vi "Acquisition Message Loop.vi"(6 "Data-Chart-Reference":refnum<vi>, 8 "error in (no error)":errorcluster, 9 "Data Queue":refnum<queue>, 10 "Data Notifier":refnum<notifier>, 11 "Message Queues":T1) -> (0 "error out":errorcluster)   [LabVIEW 2018, in "Acquisition.lvlib"]
doc: "Message loop for handling messages pertaining to the acquisition of data from the hardware."
uses:
  Acquisition.lvlib
  support/Message Queue/All Message Queues.ctl
  support/Message Queue/Message Cluster.ctl
  Hardware Configuration.ctl
  Acquisition State.ctl
  <vilib>/Platform/TimedLoop/XDataNode/timing_clust.ctl
  <vilib>/Platform/TimedLoop/XDataNode/nitl_modes.ctl
  <vilib>/Platform/TimedLoop/XDataNode/wakeup.ctl
  support/Message Queue/Enqueue Message (Single).vi
  <vilib>/Utility/error.llb/Error Cluster From Error Code.vi
  <vilib>/platform/TimedLoop/XDataNode/XDataNode.xnode
  <vilib>/ErrorRing/Error Ring.xnode
  support/Message Queue/Message Queue.lvlib
  <vilib>/Platform/TimedLoop/XDataNode/XDNodeRunTimeDep.lvlib
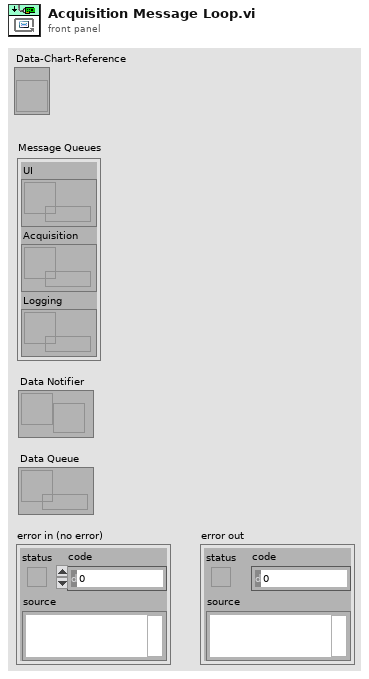
[diagram p1: front panel]
types:
  T1 = typedef "Message Queue.lvlib/All Message Queues.ctl" = cluster{"UI":refnum<queue>, "Acquisition":refnum<queue>, "Logging":refnum<queue>}
  T2 = typedef "Acquisition.lvlib/Hardware Configuration.ctl" = cluster{"DAQmx Channel 1":tag, "DAQmx Channel 2":tag, "DAQmx Channel 3":tag, "Channel 1 Name":string, "Channel 2 Name":string, "Channel 3 Name":string, "Input Config Channel 1":i32, "Input Config Channel 2":i32, "Input Config Channel 3":i32, "Offset Channel 1":dbl, "Offset Channel 2":dbl, "Offset Channel 3":dbl, "Scale Channel 1":dbl, "Scale Channel 2":dbl, "Scale Channel 3":dbl, "DAQmx Counter Channel":tag, "Counter Name":string, "Sample time":u32, "Samples per second":dbl, "Sample mode":u16, "Samples per channel":i32, "DAQmx AI Task":refnum<k21>, "DAQmx Counter Task":refnum<k21>}
  T3 = typedef "XDNodeRunTimeDep.lvlib/timing_clust.ctl" = cluster{"Expected End [f-1]":u64, "Actual End [f-1]":u64, "Finished Late? [f-1]":bool, "Expected End [i-1]":u64, "Actual End [i-1]":u64, "Finished Late? [i-1]":bool, "Expected Start [i]":u64, "Actual Start [i]":u64, "Expected Start [f]":u64, "Actual Start [f]":u64, "Source Name":string, "Structure Name":string, "Period":i64, "Deadline":i64, "Offset":i64, "Start":i64, "Priority":i32, "Timeout":i32, "Mode":T4, "Wakeup Reason":T5, "Error":errorcluster, "Source Type":string, "Secondary Source Type":string, "Global End Time":u64, "Global Start Time":u64, "Frame Duration":u64, "Iteration Duration":u64, "Assigned CPU":i32, "I/O Scan Engine Mode":u32}
  T4 = typedef "XDNodeRunTimeDep.lvlib/nitl_modes.ctl" = enum32{"No Change", "Process missed periods, maintain original phase", "Discard missed periods, maintain original phase", "Process missed periods, ignore original phase", "Discard missed periods, ignore original phase"}
  T5 = typedef "XDNodeRunTimeDep.lvlib/wakeup.ctl" = enum32{"Normal", "Aborted", "Asynchronous wakeup", "Timing source error", "Timed loop error", "Timeout"}
  T6 = typedef "Acquisition.lvlib/Acquisition State.ctl" = enum16{"Idle", "Acquiring"}
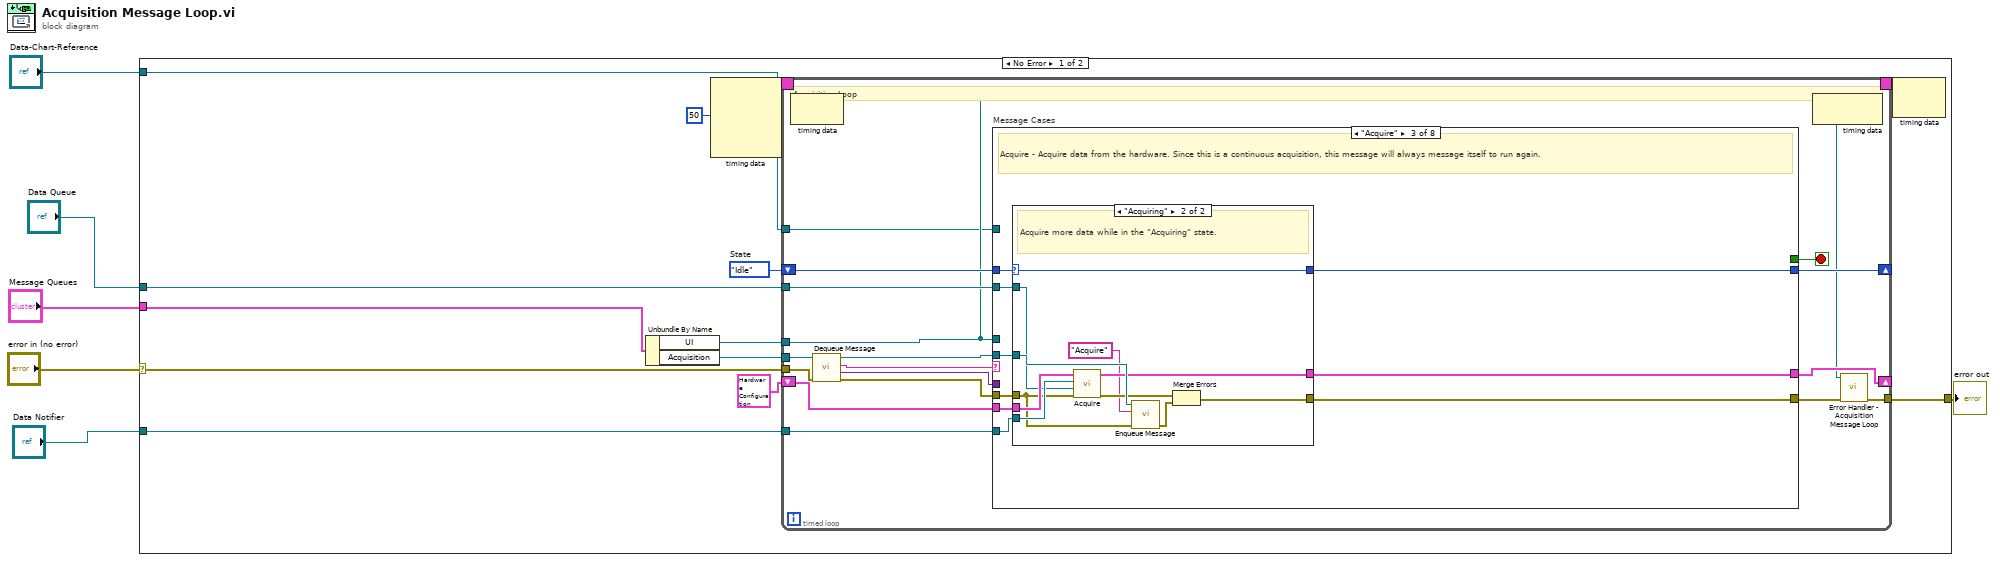
[diagram p0: block diagram]
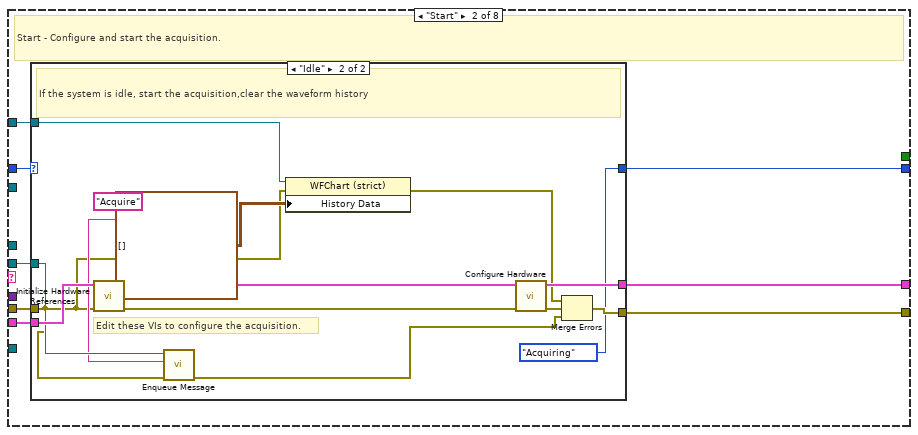
[diagram p3: hidden frame]
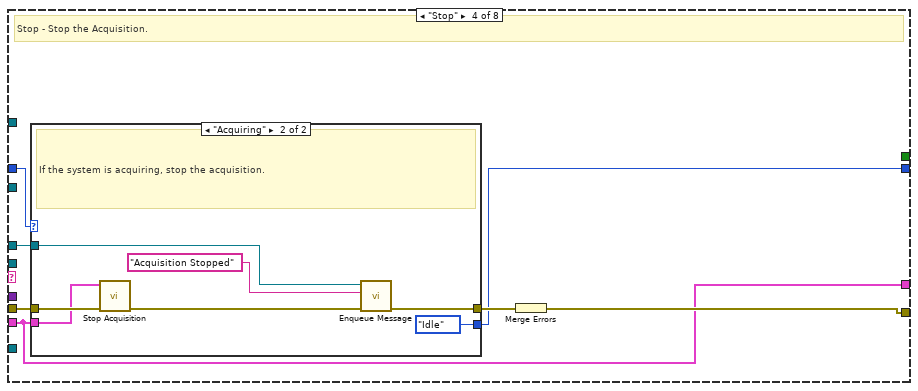
[diagram p6: hidden frame]
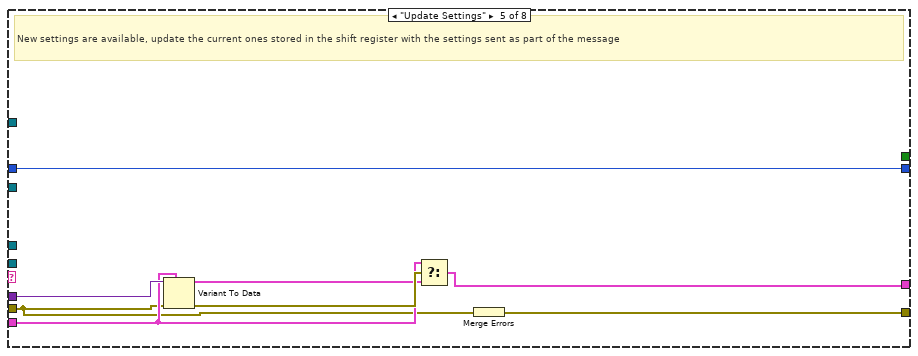
[diagram p8: hidden frame]
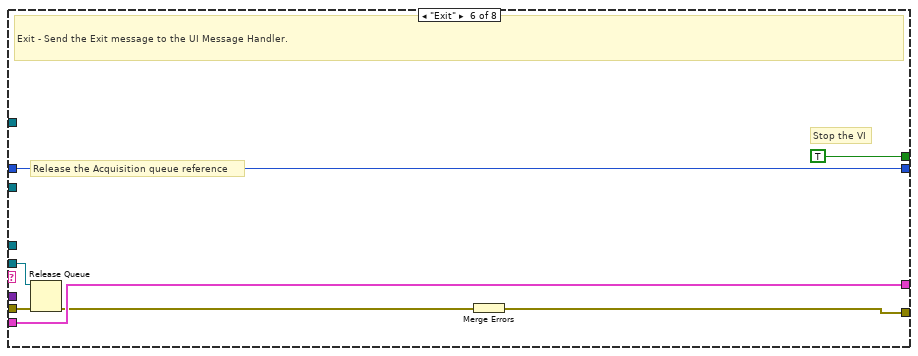
[diagram p9: hidden frame]
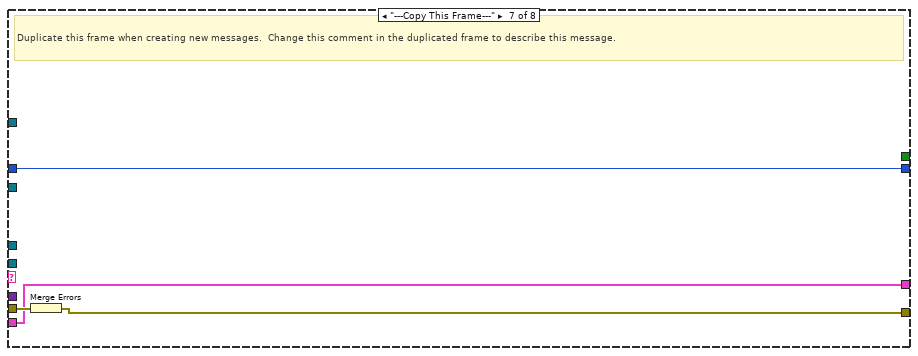
[diagram p10: hidden frame]
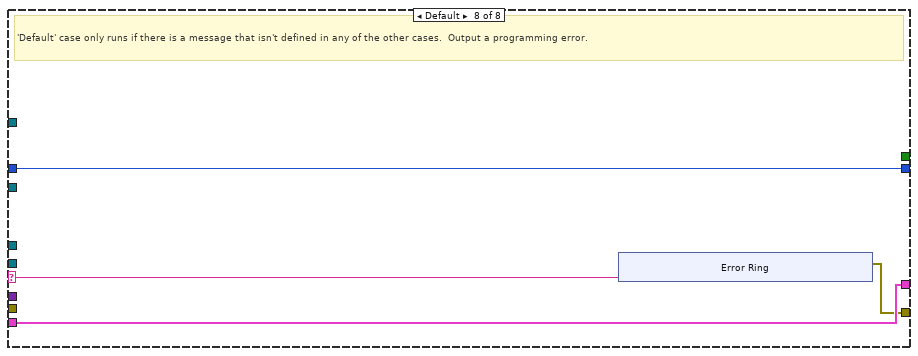
[diagram p11: hidden frame]
diagram:
  n1 = case shown="No Error" "error in (no error)" {
    selector: "error in (no error)" -> [w15 w140]
    tunnel: "Message Queues" -> [w19 _]
    tunnel: [w17 w140] -> w5
    tunnel: "Data Notifier" -> [w13 _]
    tunnel: "Data Queue" -> [w12 _]
    tunnel: "Data-Chart-Reference" -> [w10 _]
    frame No Error {
      w11 = Acquisition_State."Idle"  # State
      n2 = Unbundle By Name(w19) -> ("UI"=w14:refnum<queue>, "Acquisition"=w18:refnum<queue>)
      n3 = node-c288(i64 50 ("Period")) -> (w9:T3)  [unwired: 3 in]
      n4 = timed-loop {
        tunnel: w18 -> [w29]
        shift-right: [w35] -> _
        shift-left: T2 {"DAQmx Channel 1"="", "DAQmx Channel 2"="", "DAQmx Channel 3"="", "Channel 1 Name"="Battery Voltage", "Channel 2 Name"="Battery Current", "Channel 3 Name"="Brake torque", "Input Config Channel 1"=-1, "Input Config Channel 2"=-1, "Input Config Channel 3"=-1, "Offset Channel 1"=0.0, "Offset Channel 2"=0.0, "Offset Channel 3"=0.0, "Scale Channel 1"=0.0, "Scale Channel 2"=0.0, "Scale Channel 3"=0.0, "DAQmx Counter Channel"="", "Counter Name"="", "Sample time"=50, "Samples per second"=1000.0, "Sample mode"=0, "Samples per channel"=0, "DAQmx AI Task"="", "DAQmx Counter Task"=""} ("Data Cluster") -> [w36]
        tunnel: w14 -> [w21]
        tunnel: w13 -> [w28]
        tunnel: w12 -> [w27]
        shift-right: [w25] -> _
        shift-left: w11 -> [w26]
        tunnel: w15 -> [w33]
        tunnel: [w24] -> w17
        tunnel: w10 -> [w20]
        timing: w9 -> [_]
        timing-out: [_] -> w8
        stop <- w34 stop-if-true
        # "Acquisition Loop"
        n5 = node-c288() -> ()  [unwired: 1 in, 1 out]
        n6 = call "Dequeue Message.vi"("error in (no error)"=w33, "Message Queue"=w29) -> ("error out"=w32:errorcluster, "Message Data"=w30:variant, "Message"=w31:string, "dup Message Queue"=w22:refnum<queue>)  [unwired: 6 in]
        n7 = case "Message Cases" shown="\"Acquire\"" w31 {
          selector: w31 -> [_ _ _ _ _ _ _ w125]
          tunnel: w22 -> [_ w46 w74 _ _ w115 _ _]
          tunnel: w32 -> [w41 w47 w73 w95 w107 w117 w124 _]
          tunnel: [w41 w49 w75 w96 w113 w119 w122 w126] -> w23
          tunnel: w36 -> [w40 w48 w71 w93 w109 w118 w123 w128]
          tunnel: [w40 w45 w72 w93 w108 w118 w123 w128] -> w35
          tunnel: [_ _ _ _ _ TRUE _ _] -> w34
          tunnel: w30 -> [_ _ _ _ w112 _ _ _]
          tunnel: w21 -> [_ _ _ w90 _ _ _ _]
          tunnel: w28 -> [_ _ w70 _ _ _ _ _]
          tunnel: w27 -> [_ _ w69 _ _ _ _ _]
          tunnel: w26 -> [w39 w43 w67 w92 w106 w114 w121 w127]
          tunnel: [w39 w44 w68 w91 w106 w114 w121 w127] -> w25
          tunnel: w20 -> [_ w42 _ _ _ _ _ _]
          frame "Initialize" {
            # "Initialize  - Initialize is currently a no-op.  The hardware initialization takes place in the 'Start' message."
          }
          frame "Start" {
            # "Start - Configure and start the acquisition."
            n8 = case shown="\"Idle\"" w43 {
              selector: w43 -> [w50 _]
              tunnel: [w51 w66] -> w49
              tunnel: w48 -> [w52 w65]
              tunnel: w47 -> [w51 w55]
              tunnel: w46 -> [_ w63]
              tunnel: [w52 w60] -> w45
              tunnel: [w50 Acquisition_State."Acquiring" ("Acquisition State")] -> w44
              tunnel: w42 -> [_ w53]
              frame "Acquiring" {
                # "The system is already acquiring. Ignore the \"Start\" message."
              }
              frame "Idle" {
                # "Edit these VIs to configure the acquisition."
                # "If the system is idle, start the acquisition,clear the waveform history"
                n9 = call "Initialize Hardware References.vi"("error in (no error)"=w55, "Hardware Resources in"=w65) -> ("error out"=w62:errorcluster, "Hardware Resources out"=w57:T2)  [unwired: 8 in]
                n10 = call-poly "Enqueue Message.vi"("error in (no error)"=w55, "Message"="Acquire", "Message Queue"=w63) -> ("error out"=w64:errorcluster)  [unwired: 7 in, 1 out]
                n11 = property class="WFChart (strict)"(reference=w53, error in=w55, "History Data"=waveform(dbl)[][] []) -> (error out=w54:errorcluster)  [unwired: 1 out]
                n12 = call "Configure Hardware.vi"("error in (no error)"=w62, "Hardware Resources in"=w57) -> ("error out"=w61:errorcluster, "Hardware Resources out"=w60:T2)  [unwired: 8 in]
                n13 = Merge Errors(w54, w61, w64) -> (w66:errorcluster)
              }
            }
          }
          frame "Acquire" {
            # "Acquire - Acquire data from the hardware. Since this is a continuous acquisition, this message will always message itself to run again."
            n14 = case shown="\"Acquiring\"" w67 {
              selector: w67 -> [w76 w80]
              tunnel: [w77 w89] -> w75
              tunnel: w74 -> [_ w87]
              tunnel: w73 -> [w77 w79]
              tunnel: [w78 w85] -> w72
              tunnel: w71 -> [w78 w84]
              tunnel: w70 -> [_ w82]
              tunnel: w69 -> [_ w81]
              tunnel: [w76 w80] -> w68
              frame "Idle" {
                # "Ignore \"Acquire\" messages when the acquisition is idle."
              }
              frame "Acquiring" {
                # "Acquire more data while in the \"Acquiring\" state."
                n15 = call "Acquire.vi"("error in (no error)"=w79, "Data Queue"=w81, "Data Notifier"=w82, "Hardware Resources in"=w84) -> ("error out"=w86:errorcluster, "Hardware Resources out"=w85:T2)  [unwired: 6 in]
                n16 = call-poly "Enqueue Message.vi"("error in (no error)"=w79, "Message"="Acquire", "Message Queue"=w87) -> ("error out"=w88:errorcluster)  [unwired: 7 in, 1 out]
                n17 = Merge Errors(w86, w88) -> (w89:errorcluster)
              }
            }
          }
          frame "Stop" {
            # "Stop - Stop the Acquisition."
            n18 = case shown="\"Acquiring\"" w92 {
              selector: w92 -> [w97 _]
              tunnel: w95 -> [w98 w105]
              tunnel: [w98 w101] -> w94
              tunnel: w93 -> [_ w103]
              tunnel: [w97 Acquisition_State."Idle" ("State")] -> w91
              tunnel: w90 -> [_ w100]
              frame "Idle" {
                # "The system is already idle. Ignore the \"Stop\" message."
              }
              frame "Acquiring" {
                # "If the system is acquiring, stop the acquisition."
                n19 = call "Stop Acquisition.vi"("error in (no error)"=w105, "Hardware Resources in"=w103) -> ("error out"=w104:errorcluster)  [unwired: 9 in]
                n20 = call-poly "Enqueue Message.vi"("error in (no error)"=w104, "Message"="Acquisition Stopped", "Message Queue"=w100) -> ("error out"=w101:errorcluster)  [unwired: 7 in, 1 out]
              }
            }
            n21 = Merge Errors(w94) -> (w96:errorcluster)
          }
          frame "Update Settings" {
            # "New settings are available, update the current ones stored in the shift register with the settings sent as part of the message"
            n22 = Variant To Data(error in=w107, type=w109, Variant=w112) -> (data=w110:T2, error out=w111:errorcluster)
            n23 = Select(t=w109, s=w111, f=w110) -> (s? t:f=w108:T2)
            n24 = Merge Errors(w107) -> (w113:errorcluster)
          }
          frame "Exit" {
            # "Release the Acquisition queue reference"
            # "Stop the VI"
            # "Exit - Send the Exit message to the UI Message Handler."
            n25 = Release Queue(queue=w115, error in (no error)=w117) -> (error out=w116:errorcluster)  [unwired: 1 in, 2 out]
            n26 = Merge Errors(w116) -> (w119:errorcluster)
          }
          frame "---Copy This Frame---" {
            # "Duplicate this frame when creating new messages.  Change this comment in the duplicated frame to describe this message."
            n27 = Merge Errors(w124) -> (w122:errorcluster)
          }
          frame Default {
            # "'Default' case only runs if there is a message that isn't defined in any of the other cases.  Output a programming error."
            n28 = xnode "Error Ring"("parameter 0"=w125) -> ("error out"=w126:errorcluster)
          }
        }
        n29 = node-c288() -> ()  [unwired: 1 in, 1 out]
        n30 = call "Error Handler - Acquisition Message Loop.vi"("error in (no error)"=w23, "Message Queue"=w21) -> ("dup error in"=w24:errorcluster)  [unwired: 8 in, 1 out]
      }
      n31 = node-c288(w8) -> ()  [unwired: 1 out]
    }
    frame Error {
    }
  }
  "error out" <- w5
